vi "Global_SM Write_Data Out.vi"() -> ()   [LabVIEW 2017, in "Claw.lvlib"]
uses:
  Claw.lvlib
  <vilib>/Rock Robotics/WPI/Solenoid/WPI_SolenoidValue.ctl
  _SHARE ALL/TypeDef Share All/CLUSTER_TalonInput.ctl
  System Drivers/Phoenix-LabVIEW/Motor Controller/Controls/CTRE_Phoenix_MotorControl_ControlMode.ctl
  _SHARE ALL/RoboRio Share All/SRX Share All/TypeDefs SRX/Cluster_SRX_PIDF.ctl
panel:
  in  "Claw_SM_Right_Claw":T1 {"Talon Mode" items=["PercentOutput"=0, "Position"=1, "Velocity"=2, "Current"=3, "Follower"=5, "MotionProfile"=6, "MotionMagic"=7, "MotionMagicArc"=8, "MotionProfileArc"=10, "Disabled"=15]}
  in  "Claw_SM_Left_Claw":T1 {"Talon Mode" items=["PercentOutput"=0, "Position"=1, "Velocity"=2, "Current"=3, "Follower"=5, "MotionProfile"=6, "MotionMagic"=7, "MotionMagicArc"=8, "MotionProfileArc"=10, "Disabled"=15]}
  in  "Claw_SM_Pistion_Input":T4
  # "The Names of the Data items in the Global Variable MUST describe who the Single Writer is\nNaming Convention of all Data Items is:   \nLib Name_Loop Name (SM or SEN or ACT)_Data Name\nExamples:\nDrive_ACT_X axis\nGameController_SEN_JoystickLeft\nHopper_SM_AgitatorSpeed"
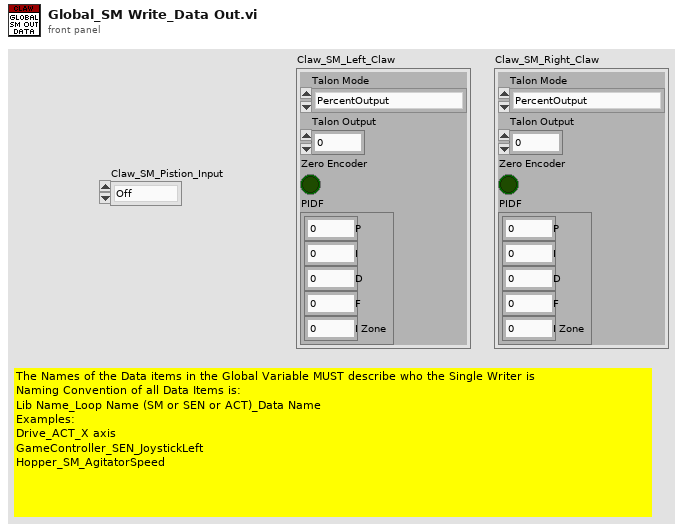
[diagram p1: front panel]
types:
  T1 = typedef "CLUSTER_TalonInput.ctl" = cluster{"Talon Mode":T2, "Talon Output":dbl, "Zero Encoder":bool, "PIDF":T3}
  T2 = typedef "CTRE_Phoenix_MotorControl_ControlMode.ctl" = u16
  T3 = typedef "Cluster_SRX_PIDF.ctl" = cluster{"P":dbl, "I":dbl, "D":dbl, "F":dbl, "I Zone":dbl}
  T4 = typedef "WPI_SolenoidValue.ctl" = enum16{"Off", "On", "Forward", "Reverse"}
diagram:
